vi "Set SshHostKeyFingerprint.vi"(8 "error in (no error)":errorcluster, 10 "SshHostKeyFingerprint":string, 11 "SessionOptions-SCP in":refnum<class "SessionOptions-SCP.lvclass">) -> (0 "error out":errorcluster, 3 "SessionOptions-SCP out":refnum<class "SessionOptions-SCP.lvclass">)   [LabVIEW 2015, in "WinSCP.lvlib" / "SessionOptions-SCP.lvclass"]
uses:
  SessionOptions-SCP.lvclass
  SessionOptions-SCP.lvclass/SessionOptions-SCP.ctl
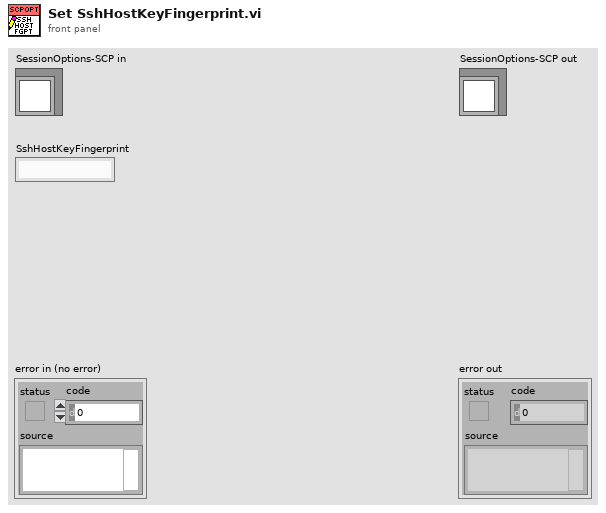
[diagram p1: front panel]
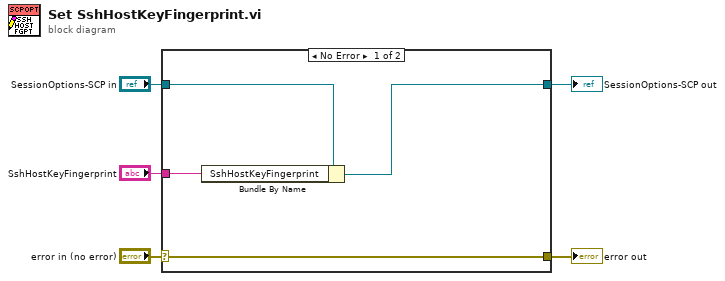
[diagram p0: block diagram]
diagram:
  n1 = case shown="No Error" "error in (no error)" {
    selector: "error in (no error)" -> [w6 w10]
    tunnel: [w6 w10] -> w4
    tunnel: [w7 w11] -> w2
    tunnel: "SessionOptions-SCP in" -> [w9 w11]
    tunnel: "SshHostKeyFingerprint" -> [w8 _]
    frame No Error {
      n2 = Bundle By Name(cluster=w9, "SshHostKeyFingerprint"=w8) -> (w7:refnum<class "SessionOptions-SCP.lvclass">)
    }
    frame Error {
    }
  }
  "error out" <- w4
  "SessionOptions-SCP out" <- w2
